vi "read_plc_global.vi"() -> ()   [LabVIEW 2011]
panel:
  out "Error in AO PLCs":errorcluster
  out "Error in AI PLCs":errorcluster
  out "LB201_B230_SV201":string
  out "LB201_B230_SV401":string
  out "LB201_B230_ST902":string
  out "LB201_B230_ST901":string
  out "LB201_A213_ST902":string
  out "LB201_A213_ST901":string
  out "LB201_A235_SV401":string
  out "LB201_A235_SV201":string
  out "LB201_A235_ST902":string
  out "LB201_A235_ST901":string
  out "LB201_A225_SV401":string
  out "LB201_A225_SV201":string
  out "LB201_A225_ST902":string
  out "LB201_A225_ST901":string
  out "LB201_A213_SV201":string
  out "LB201_A213_ST401":string
  out "LB201_B230_GQ101":string
  out "LB201_B230_GT101":string
  out "LB201_B226_GT301":string
  out "LB201_A235_GQ101":string
  out "LB201_A235_GT101":string
  out "LB201_B230_GN501":string
  out "LB201_A235_GN501":string
  out "LB201_A225_GT101":string
  out "LB201_A225_GQ101":string
  out "LB201_A225_GN501":string
  out "LB201_A213_GT101":string
  out "LB201_A213_GQ101":string
  out "LB201_A213_GN501":string
  out "Deque error":errorcluster
  out "DataSocket error":errorcluster
  out "# Sent Data":u64
  in  "Version":string
  in  "UpTime":string
  in  "StartupTime":string
  in  "ElapsedTime":u32
  in  "Command":string
  # "OPC Server Status"
  # "AI PLCs"
  # "AO PLCs"
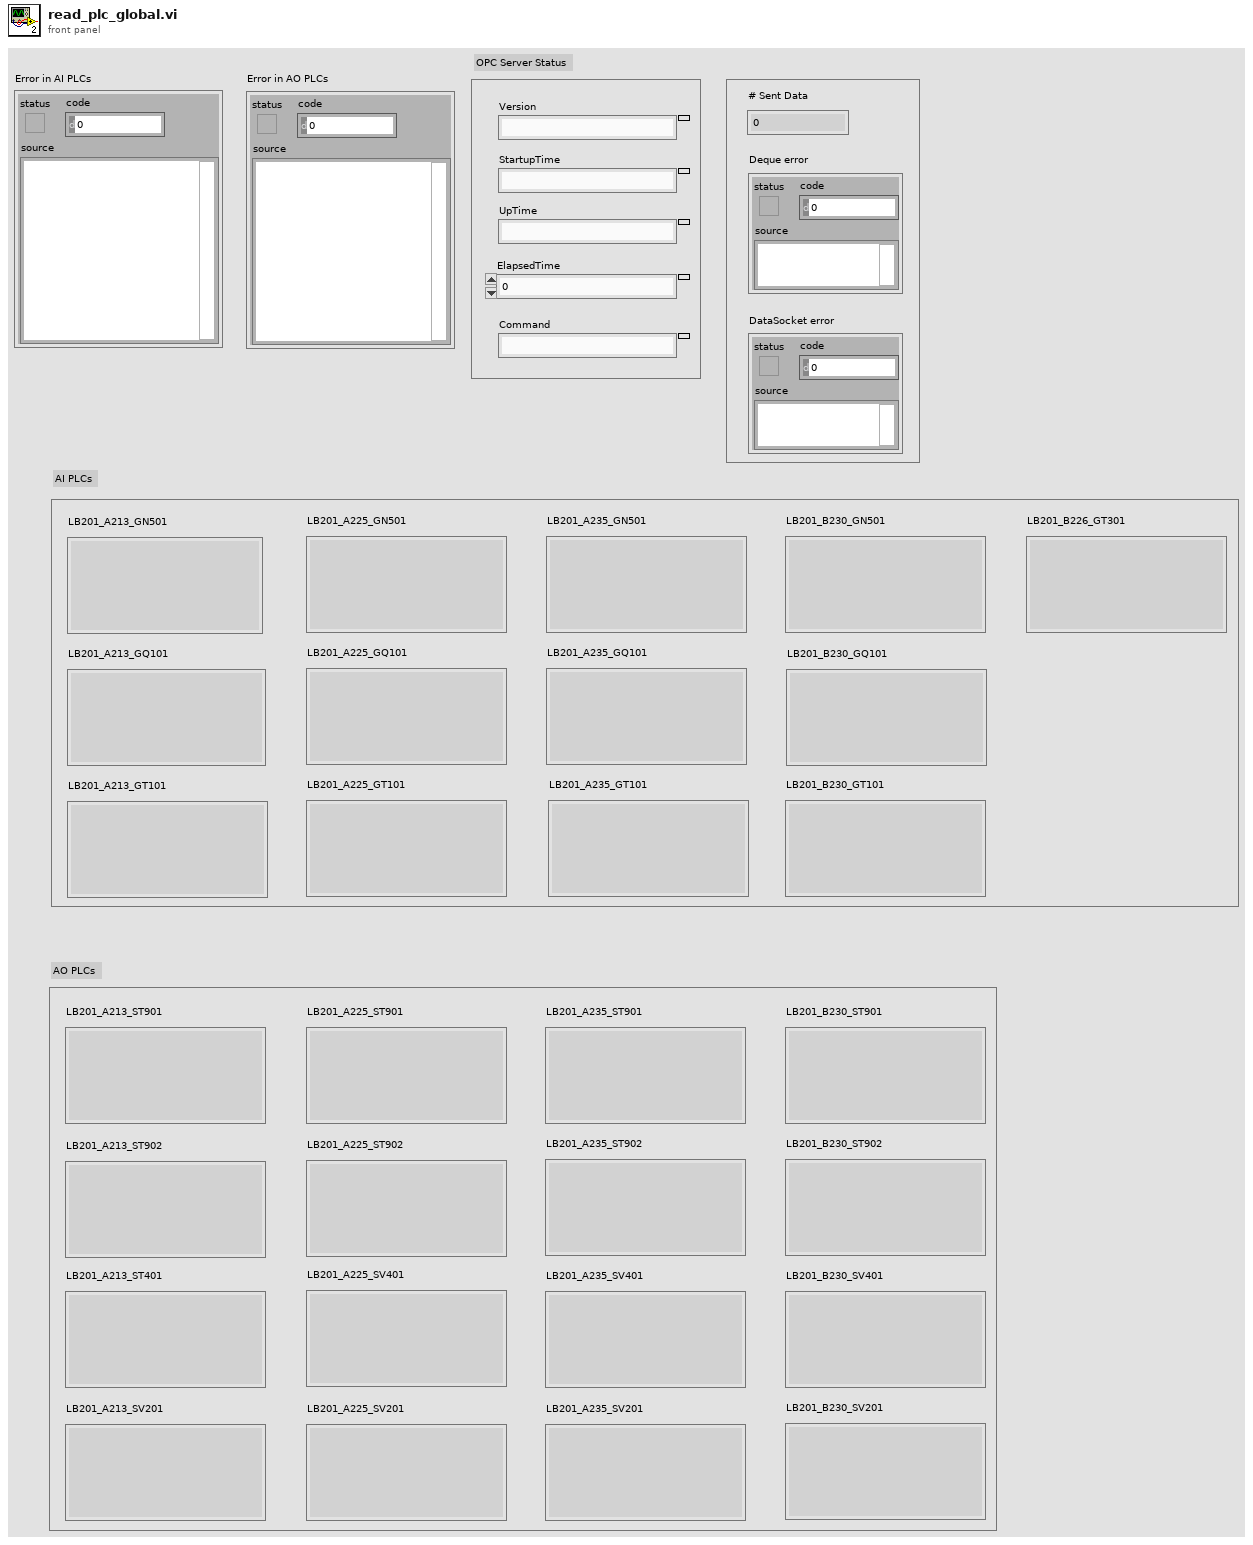
[diagram p1: front panel]
types:
  T1 = enum16{"Read", "Write", "ReadWrite", "BufferedRead", "BufferedReadWrite"}
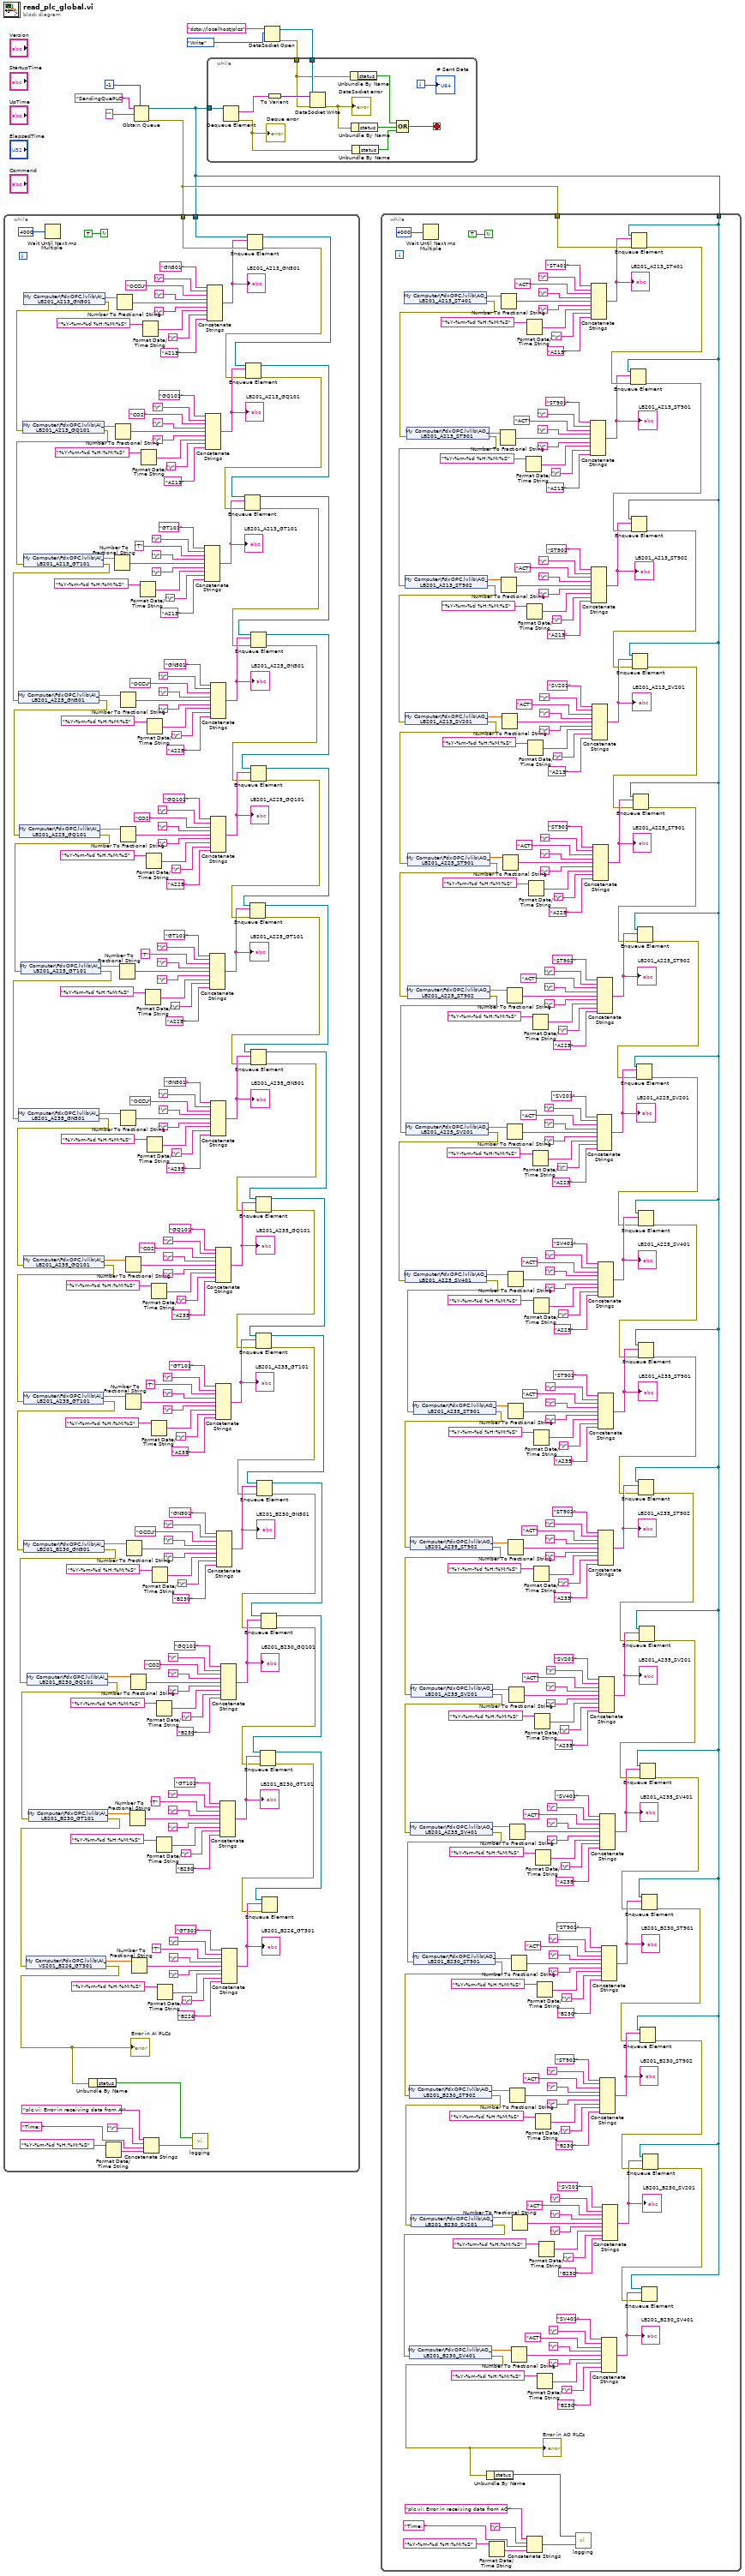
[diagram p0: block diagram]
diagram:
  n1 = Obtain Queue(max queue size (-1, unlimited)=-1, name (unnamed)="SendingQuePLC", element data type="") -> (queue out=w1:refnum<queue>, error out=w2:errorcluster)  [unwired: 2 in, 1 out]
  n2 = while {
    tunnel: w2 -> [w212]
    tunnel: w1 -> [w211]
    stop <- TRUE continue-if-true
    n3 = shared-variable "My Computer\\FdxOPC.lvlib\\AI_LB201_A213_GN501"() -> (w172:sgl, error out=w29:errorcluster)  [unwired: 1 in]
    n4 = shared-variable "My Computer\\FdxOPC.lvlib\\AI_LB201_A213_GQ101"(error in=w29) -> (w171:sgl, error out=w28:errorcluster)
    n5 = shared-variable "My Computer\\FdxOPC.lvlib\\AI_LB201_A213_GT101"(error in=w28) -> (w170:sgl, error out=w27:errorcluster)
    n6 = shared-variable "My Computer\\FdxOPC.lvlib\\AI_LB201_A225_GN501"(error in=w27) -> (w59:sgl, error out=w26:errorcluster)
    n7 = shared-variable "My Computer\\FdxOPC.lvlib\\AI_LB201_A225_GQ101"(error in=w26) -> (w56:sgl, error out=w25:errorcluster)
    n8 = shared-variable "My Computer\\FdxOPC.lvlib\\AI_LB201_A225_GT101"(error in=w25) -> (w55:sgl, error out=w24:errorcluster)
    n9 = shared-variable "My Computer\\FdxOPC.lvlib\\AI_LB201_A235_GN501"(error in=w24) -> (w54:sgl, error out=w23:errorcluster)
    n10 = shared-variable "My Computer\\FdxOPC.lvlib\\AI_LB201_A235_GQ101"(error in=w23) -> (w53:sgl, error out=w22:errorcluster)
    n11 = shared-variable "My Computer\\FdxOPC.lvlib\\AI_LB201_A235_GT101"(error in=w22) -> (w52:sgl, error out=w21:errorcluster)
    n12 = shared-variable "My Computer\\FdxOPC.lvlib\\AI_LB201_B230_GN501"(error in=w21) -> (w51:sgl, error out=w20:errorcluster)
    n13 = shared-variable "My Computer\\FdxOPC.lvlib\\AI_LB201_B230_GQ101"(error in=w20) -> (w50:sgl, error out=w19:errorcluster)
    n14 = shared-variable "My Computer\\FdxOPC.lvlib\\AI_LB201_B230_GT101"(error in=w19) -> (w49:sgl, error out=w18:errorcluster)
    n15 = shared-variable "My Computer\\FdxOPC.lvlib\\AI_VS201_B226_GT301"(error in=w18) -> (w48:sgl, error out=w17:errorcluster)
    "Error in AI PLCs" <- w17
    n16 = Wait Until Next ms Multiple(millisecond multiple=u32 4000) -> ()  [unwired: 1 out]
    n17 = Unbundle By Name(w17) -> ("status"=w10:bool)
    n18 = Format Date/Time String(time format string (%c)="%Y-%m-%d %H:%M:%S") -> (date/time string=w12:string)  [unwired: 2 in]
    n19 = Number To Fractional String(number=w170) -> (F-format string=w183:string)  [unwired: 3 in]
    n20 = Number To Fractional String(number=w171) -> (F-format string=w192:string)  [unwired: 3 in]
    n21 = Number To Fractional String(number=w172) -> (F-format string=w205:string)  [unwired: 3 in]
    n22 = Number To Fractional String(number=w55) -> (F-format string=w143:string)  [unwired: 3 in]
    n23 = Number To Fractional String(number=w56) -> (F-format string=w152:string)  [unwired: 3 in]
    n24 = Number To Fractional String(number=w59) -> (F-format string=w165:string)  [unwired: 3 in]
    n25 = Number To Fractional String(number=w54) -> (F-format string=w130:string)  [unwired: 3 in]
    n26 = Number To Fractional String(number=w52) -> (F-format string=w108:string)  [unwired: 3 in]
    n27 = Number To Fractional String(number=w53) -> (F-format string=w99:string)  [unwired: 3 in]
    n28 = Number To Fractional String(number=w51) -> (F-format string=w121:string)  [unwired: 3 in]
    n29 = Number To Fractional String(number=w49) -> (F-format string=w77:string)  [unwired: 3 in]
    n30 = Number To Fractional String(number=w50) -> (F-format string=w86:string)  [unwired: 3 in]
    n31 = Number To Fractional String(number=w48) -> (F-format string=w64:string)  [unwired: 3 in]
    n32 = Format Date/Time String(time format string (%c)="%Y-%m-%d %H:%M:%S") -> (date/time string=w182:string)  [unwired: 2 in]
    n33 = Format Date/Time String(time format string (%c)="%Y-%m-%d %H:%M:%S") -> (date/time string=w193:string)  [unwired: 2 in]
    n34 = Format Date/Time String(time format string (%c)="%Y-%m-%d %H:%M:%S") -> (date/time string=w204:string)  [unwired: 2 in]
    n35 = Concatenate Strings("plc.vi: Error in receiving data from AI", "\r", "Time: ", w12) -> (w13:string)
    n36 = Format Date/Time String(time format string (%c)="%Y-%m-%d %H:%M:%S") -> (date/time string=w142:string)  [unwired: 2 in]
    n37 = Format Date/Time String(time format string (%c)="%Y-%m-%d %H:%M:%S") -> (date/time string=w153:string)  [unwired: 2 in]
    n38 = Format Date/Time String(time format string (%c)="%Y-%m-%d %H:%M:%S") -> (date/time string=w164:string)  [unwired: 2 in]
    n39 = Format Date/Time String(time format string (%c)="%Y-%m-%d %H:%M:%S") -> (date/time string=w131:string)  [unwired: 2 in]
    n40 = Format Date/Time String(time format string (%c)="%Y-%m-%d %H:%M:%S") -> (date/time string=w109:string)  [unwired: 2 in]
    n41 = Format Date/Time String(time format string (%c)="%Y-%m-%d %H:%M:%S") -> (date/time string=w98:string)  [unwired: 2 in]
    n42 = Format Date/Time String(time format string (%c)="%Y-%m-%d %H:%M:%S") -> (date/time string=w120:string)  [unwired: 2 in]
    n43 = Format Date/Time String(time format string (%c)="%Y-%m-%d %H:%M:%S") -> (date/time string=w76:string)  [unwired: 2 in]
    n44 = Format Date/Time String(time format string (%c)="%Y-%m-%d %H:%M:%S") -> (date/time string=w87:string)  [unwired: 2 in]
    n45 = Format Date/Time String(time format string (%c)="%Y-%m-%d %H:%M:%S") -> (date/time string=w65:string)  [unwired: 2 in]
    n46 = call "logging.vi"("Body"=w13, "Enable"=w10) -> ()  [unwired: 1 in]
    n47 = Concatenate Strings("GT101" ("string"), "\r", "T" ("string"), "\r", w183, "\r", w182, "\r", "A213") -> (w186:string)
    "LB201_A213_GT101" <- w186
    n48 = Concatenate Strings("GQ101" ("string"), "\r", "CO2" ("string"), "\r", w192, "\r", w193, "\r", "A213") -> (w189:string)
    "LB201_A213_GQ101" <- w189
    n49 = Concatenate Strings("GN501" ("string"), "\r", "OCCU" ("string"), "\r", w205, "\r", w204, "\r", "A213") -> (w210:string)
    "LB201_A213_GN501" <- w210
    n50 = Concatenate Strings("GT101" ("string"), "\r", "T" ("string"), "\r", w143, "\r", w142, "\r", "A225") -> (w146:string)
    "LB201_A225_GT101" <- w146
    n51 = Concatenate Strings("GQ101" ("string"), "\r", "CO2" ("string"), "\r", w152, "\r", w153, "\r", "A225") -> (w149:string)
    "LB201_A225_GQ101" <- w149
    n52 = Concatenate Strings("GN501" ("string"), "\r", "OCCU" ("string"), "\r", w165, "\r", w164, "\r", "A225") -> (w168:string)
    "LB201_A225_GN501" <- w168
    n53 = Concatenate Strings("GN501" ("string"), "\r", "OCCU" ("string"), "\r", w130, "\r", w131, "\r", "A235") -> (w127:string)
    "LB201_A235_GN501" <- w127
    n54 = Concatenate Strings("GT101" ("string"), "\r", "T" ("string"), "\r", w108, "\r", w109, "\r", "A235") -> (w105:string)
    "LB201_A235_GT101" <- w105
    n55 = Concatenate Strings("GQ101" ("string"), "\r", "CO2" ("string"), "\r", w99, "\r", w98, "\r", "A235") -> (w102:string)
    "LB201_A235_GQ101" <- w102
    n56 = Concatenate Strings("GN501" ("string"), "\r", "OCCU" ("string"), "\r", w121, "\r", w120, "\r", "B230") -> (w124:string)
    "LB201_B230_GN501" <- w124
    n57 = Concatenate Strings("GT101" ("string"), "\r", "T" ("string"), "\r", w77, "\r", w76, "\r", "B230") -> (w80:string)
    "LB201_B230_GT101" <- w80
    n58 = Concatenate Strings("GQ101" ("string"), "\r", "CO2" ("string"), "\r", w86, "\r", w87, "\r", "B230") -> (w83:string)
    "LB201_B230_GQ101" <- w83
    n59 = Concatenate Strings("GT301" ("string"), "\r", "T" ("string"), "\r", w64, "\r", w65, "\r", "B226") -> (w61:string)
    "LB201_B226_GT301" <- w61
    n60 = Enqueue Element(queue=w211, element=w210, error in (no error)=w212) -> (queue out=w176:refnum<queue>, error out=w174:errorcluster)  [unwired: 1 in, 1 out]
    n61 = Enqueue Element(queue=w176, element=w189, error in (no error)=w174) -> (queue out=w175:refnum<queue>, error out=w173:errorcluster)  [unwired: 1 in, 1 out]
    n62 = Enqueue Element(queue=w175, element=w186, error in (no error)=w173) -> (queue out=w58:refnum<queue>, error out=w57:errorcluster)  [unwired: 1 in, 1 out]
    n63 = Enqueue Element(queue=w58, element=w168, error in (no error)=w57) -> (queue out=w47:refnum<queue>, error out=w46:errorcluster)  [unwired: 1 in, 1 out]
    n64 = Enqueue Element(queue=w47, element=w149, error in (no error)=w46) -> (queue out=w45:refnum<queue>, error out=w44:errorcluster)  [unwired: 1 in, 1 out]
    n65 = Enqueue Element(queue=w45, element=w146, error in (no error)=w44) -> (queue out=w43:refnum<queue>, error out=w42:errorcluster)  [unwired: 1 in, 1 out]
    n66 = Enqueue Element(queue=w43, element=w127, error in (no error)=w42) -> (queue out=w41:refnum<queue>, error out=w40:errorcluster)  [unwired: 1 in, 1 out]
    n67 = Enqueue Element(queue=w41, element=w102, error in (no error)=w40) -> (queue out=w39:refnum<queue>, error out=w38:errorcluster)  [unwired: 1 in, 1 out]
    n68 = Enqueue Element(queue=w39, element=w105, error in (no error)=w38) -> (queue out=w37:refnum<queue>, error out=w36:errorcluster)  [unwired: 1 in, 1 out]
    n69 = Enqueue Element(queue=w37, element=w124, error in (no error)=w36) -> (queue out=w35:refnum<queue>, error out=w34:errorcluster)  [unwired: 1 in, 1 out]
    n70 = Enqueue Element(queue=w35, element=w83, error in (no error)=w34) -> (queue out=w33:refnum<queue>, error out=w32:errorcluster)  [unwired: 1 in, 1 out]
    n71 = Enqueue Element(queue=w33, element=w80, error in (no error)=w32) -> (queue out=w31:refnum<queue>, error out=w30:errorcluster)  [unwired: 1 in, 1 out]
    n72 = Enqueue Element(queue=w31, element=w61, error in (no error)=w30) -> ()  [unwired: 1 in, 3 out]
  }
  n73 = DataSocket Open(10:T1."Write" ("mode"), 11:"dstp://localhost/plcs" ("URL 3")) -> (0:w4:errorcluster, 3:w5:refnum<k13>)  [unwired: 2 in]
  n74 = while {
    tunnel: w1 -> [w225]
    tunnel: w5 -> [w224]
    tunnel: w4 -> [w217]
    i -> [w214]
    stop <- w215 stop-if-true
    n75 = Dequeue Element(queue=w225) -> (element=w222:string, error out=w221:errorcluster)  [unwired: 2 in, 2 out]
    "Deque error" <- w221
    n76 = To Variant(anything=w222) -> (Variant=w223:variant)
    n77 = DataSocket Write(8:w217, 10:w223, 11:w224) -> (0:w220:errorcluster)  [unwired: 3 out]
    "DataSocket error" <- w220
    n78 = Unbundle By Name(w217) -> ("status"=w216:bool)
    n79 = Unbundle By Name(w220) -> ("status"=w219:bool)
    n80 = Unbundle By Name(w221) -> ("status"=w218:bool)
    n81 = Compound Arithmetic op=OR(w216, w219, w218) -> (w215:bool)
    "# Sent Data" <- w214
  }
  n82 = while {
    tunnel: w2 -> [w327]
    tunnel: w1 -> [w226]
    stop <- TRUE continue-if-true
    n83 = shared-variable "My Computer\\FdxOPC.lvlib\\AO_LB201_A213_ST401"() -> (w326:sgl, error out=w249:errorcluster)  [unwired: 1 in]
    n84 = shared-variable "My Computer\\FdxOPC.lvlib\\AO_LB201_A213_ST901"(error in=w249) -> (w325:sgl, error out=w248:errorcluster)
    n85 = shared-variable "My Computer\\FdxOPC.lvlib\\AO_LB201_A213_ST902"(error in=w248) -> (w324:sgl, error out=w247:errorcluster)
    n86 = shared-variable "My Computer\\FdxOPC.lvlib\\AO_LB201_A213_SV201"(error in=w247) -> (w323:sgl, error out=w246:errorcluster)
    n87 = shared-variable "My Computer\\FdxOPC.lvlib\\AO_LB201_A225_ST901"(error in=w246) -> (w319:sgl, error out=w245:errorcluster)
    n88 = shared-variable "My Computer\\FdxOPC.lvlib\\AO_LB201_A225_ST902"(error in=w245) -> (w318:sgl, error out=w244:errorcluster)
    n89 = shared-variable "My Computer\\FdxOPC.lvlib\\AO_LB201_A225_SV201"(error in=w244) -> (w317:sgl, error out=w243:errorcluster)
    n90 = shared-variable "My Computer\\FdxOPC.lvlib\\AO_LB201_A225_SV401"(error in=w243) -> (w316:sgl, error out=w242:errorcluster)
    n91 = shared-variable "My Computer\\FdxOPC.lvlib\\AO_LB201_A235_ST901"(error in=w242) -> (w309:sgl, error out=w241:errorcluster)
    n92 = shared-variable "My Computer\\FdxOPC.lvlib\\AO_LB201_A235_ST902"(error in=w241) -> (w308:sgl, error out=w240:errorcluster)
    n93 = shared-variable "My Computer\\FdxOPC.lvlib\\AO_LB201_A235_SV201"(error in=w240) -> (w307:sgl, error out=w239:errorcluster)
    n94 = shared-variable "My Computer\\FdxOPC.lvlib\\AO_LB201_A235_SV401"(error in=w239) -> (w306:sgl, error out=w238:errorcluster)
    n95 = shared-variable "My Computer\\FdxOPC.lvlib\\AO_LB201_B230_ST901"(error in=w238) -> (w258:sgl, error out=w237:errorcluster)
    n96 = shared-variable "My Computer\\FdxOPC.lvlib\\AO_LB201_B230_ST902"(error in=w237) -> (w257:sgl, error out=w236:errorcluster)
    n97 = shared-variable "My Computer\\FdxOPC.lvlib\\AO_LB201_B230_SV201"(error in=w236) -> (w256:sgl, error out=w235:errorcluster)
    n98 = shared-variable "My Computer\\FdxOPC.lvlib\\AO_LB201_B230_SV401"(error in=w235) -> (w255:sgl, error out=w234:errorcluster)
    "Error in AO PLCs" <- w234
    n99 = Wait Until Next ms Multiple(millisecond multiple=u32 4000) -> ()  [unwired: 1 out]
    n100 = Unbundle By Name(w234) -> ("status"=w227:bool)
    n101 = Format Date/Time String(time format string (%c)="%Y-%m-%d %H:%M:%S") -> (date/time string=w229:string)  [unwired: 2 in]
    n102 = Number To Fractional String(number=w325) -> (F-format string=w443:string)  [unwired: 3 in]
    n103 = Number To Fractional String(number=w326) -> (F-format string=w435:string)  [unwired: 3 in]
    n104 = Number To Fractional String(number=w324) -> (F-format string=w456:string)  [unwired: 3 in]
    n105 = Number To Fractional String(number=w323) -> (F-format string=w422:string)  [unwired: 3 in]
    n106 = Number To Fractional String(number=w319) -> (F-format string=w334:string)  [unwired: 3 in]
    n107 = Number To Fractional String(number=w317) -> (F-format string=w356:string)  [unwired: 3 in]
    n108 = Number To Fractional String(number=w318) -> (F-format string=w347:string)  [unwired: 3 in]
    n109 = Number To Fractional String(number=w316) -> (F-format string=w369:string)  [unwired: 3 in]
    n110 = Number To Fractional String(number=w308) -> (F-format string=w391:string)  [unwired: 3 in]
    n111 = Number To Fractional String(number=w309) -> (F-format string=w400:string)  [unwired: 3 in]
    n112 = Number To Fractional String(number=w307) -> (F-format string=w378:string)  [unwired: 3 in]
    n113 = Number To Fractional String(number=w306) -> (F-format string=w413:string)  [unwired: 3 in]
    n114 = Number To Fractional String(number=w257) -> (F-format string=w286:string)  [unwired: 3 in]
    n115 = Number To Fractional String(number=w258) -> (F-format string=w295:string)  [unwired: 3 in]
    n116 = Number To Fractional String(number=w255) -> (F-format string=w273:string)  [unwired: 3 in]
    n117 = Number To Fractional String(number=w256) -> (F-format string=w265:string)  [unwired: 3 in]
    n118 = Format Date/Time String(time format string (%c)="%Y-%m-%d %H:%M:%S") -> (date/time string=w444:string)  [unwired: 2 in]
    n119 = Format Date/Time String(time format string (%c)="%Y-%m-%d %H:%M:%S") -> (date/time string=w434:string)  [unwired: 2 in]
    n120 = Concatenate Strings("plc.vi: Error in receiving data from AO", "\r", "Time: ", w229) -> (w230:string)
    n121 = Format Date/Time String(time format string (%c)="%Y-%m-%d %H:%M:%S") -> (date/time string=w455:string)  [unwired: 2 in]
    n122 = Format Date/Time String(time format string (%c)="%Y-%m-%d %H:%M:%S") -> (date/time string=w423:string)  [unwired: 2 in]
    n123 = Format Date/Time String(time format string (%c)="%Y-%m-%d %H:%M:%S") -> (date/time string=w335:string)  [unwired: 2 in]
    n124 = Format Date/Time String(time format string (%c)="%Y-%m-%d %H:%M:%S") -> (date/time string=w357:string)  [unwired: 2 in]
    n125 = Format Date/Time String(time format string (%c)="%Y-%m-%d %H:%M:%S") -> (date/time string=w346:string)  [unwired: 2 in]
    n126 = Format Date/Time String(time format string (%c)="%Y-%m-%d %H:%M:%S") -> (date/time string=w368:string)  [unwired: 2 in]
    n127 = Format Date/Time String(time format string (%c)="%Y-%m-%d %H:%M:%S") -> (date/time string=w390:string)  [unwired: 2 in]
    n128 = Format Date/Time String(time format string (%c)="%Y-%m-%d %H:%M:%S") -> (date/time string=w401:string)  [unwired: 2 in]
    n129 = Format Date/Time String(time format string (%c)="%Y-%m-%d %H:%M:%S") -> (date/time string=w379:string)  [unwired: 2 in]
    n130 = Format Date/Time String(time format string (%c)="%Y-%m-%d %H:%M:%S") -> (date/time string=w412:string)  [unwired: 2 in]
    n131 = Format Date/Time String(time format string (%c)="%Y-%m-%d %H:%M:%S") -> (date/time string=w285:string)  [unwired: 2 in]
    n132 = Format Date/Time String(time format string (%c)="%Y-%m-%d %H:%M:%S") -> (date/time string=w296:string)  [unwired: 2 in]
    n133 = Format Date/Time String(time format string (%c)="%Y-%m-%d %H:%M:%S") -> (date/time string=w274:string)  [unwired: 2 in]
    n134 = Format Date/Time String(time format string (%c)="%Y-%m-%d %H:%M:%S") -> (date/time string=w264:string)  [unwired: 2 in]
    n135 = call "logging.vi"("Body"=w230, "Enable"=w227) -> ()  [unwired: 1 in]
    n136 = Concatenate Strings("ST901" ("string"), "\r", "ACT" ("string"), "\r", w443, "\r", w444, "\r", "A213") -> (w311:string)
    "LB201_A213_ST901" <- w311
    n137 = Concatenate Strings("ST401" ("string"), "\r", "ACT" ("string"), "\r", w435, "\r", w434, "\r", "A213") -> (w438:string)
    "LB201_A213_ST401" <- w438
    n138 = Concatenate Strings("ST902" ("string"), "\r", "ACT" ("string"), "\r", w456, "\r", w455, "\r", "A213") -> (w310:string)
    "LB201_A213_ST902" <- w310
    n139 = Concatenate Strings("SV201" ("string"), "\r", "ACT" ("string"), "\r", w422, "\r", w423, "\r", "A213") -> (w419:string)
    "LB201_A213_SV201" <- w419
    n140 = Concatenate Strings("ST901" ("string"), "\r", "ACT" ("string"), "\r", w334, "\r", w335, "\r", "A225") -> (w331:string)
    "LB201_A225_ST901" <- w331
    n141 = Concatenate Strings("SV201" ("string"), "\r", "ACT" ("string"), "\r", w356, "\r", w357, "\r", "A225") -> (w353:string)
    "LB201_A225_SV201" <- w353
    n142 = Concatenate Strings("ST902" ("string"), "\r", "ACT" ("string"), "\r", w347, "\r", w346, "\r", "A225") -> (w350:string)
    "LB201_A225_ST902" <- w350
    n143 = Concatenate Strings("SV401" ("string"), "\r", "ACT" ("string"), "\r", w369, "\r", w368, "\r", "A225") -> (w372:string)
    "LB201_A225_SV401" <- w372
    n144 = Concatenate Strings("ST902" ("string"), "\r", "ACT" ("string"), "\r", w391, "\r", w390, "\r", "A235") -> (w394:string)
    "LB201_A235_ST902" <- w394
    n145 = Concatenate Strings("ST901" ("string"), "\r", "ACT" ("string"), "\r", w400, "\r", w401, "\r", "A235") -> (w397:string)
    "LB201_A235_ST901" <- w397
    n146 = Concatenate Strings("SV201" ("string"), "\r", "ACT" ("string"), "\r", w378, "\r", w379, "\r", "A235") -> (w375:string)
    "LB201_A235_SV201" <- w375
    n147 = Concatenate Strings("SV401" ("string"), "\r", "ACT" ("string"), "\r", w413, "\r", w412, "\r", "A235") -> (w416:string)
    "LB201_A235_SV401" <- w416
    n148 = Concatenate Strings("ST902" ("string"), "\r", "ACT" ("string"), "\r", w286, "\r", w285, "\r", "B230") -> (w289:string)
    "LB201_B230_ST902" <- w289
    n149 = Concatenate Strings("ST901" ("string"), "\r", "ACT" ("string"), "\r", w295, "\r", w296, "\r", "B230") -> (w292:string)
    "LB201_B230_ST901" <- w292
    n150 = Concatenate Strings("SV401" ("string"), "\r", "ACT" ("string"), "\r", w273, "\r", w274, "\r", "B230") -> (w270:string)
    "LB201_B230_SV401" <- w270
    n151 = Concatenate Strings("SV201" ("string"), "\r", "ACT" ("string"), "\r", w265, "\r", w264, "\r", "B230") -> (w252:string)
    "LB201_B230_SV201" <- w252
    n152 = Enqueue Element(queue=w226, element=w438, error in (no error)=w327) -> (error out=w322:errorcluster)  [unwired: 1 in, 2 out]
    n153 = Enqueue Element(queue=w226, element=w311, error in (no error)=w322) -> (error out=w321:errorcluster)  [unwired: 1 in, 2 out]
    n154 = Enqueue Element(queue=w226, element=w310, error in (no error)=w321) -> (error out=w320:errorcluster)  [unwired: 1 in, 2 out]
    n155 = Enqueue Element(queue=w226, element=w419, error in (no error)=w320) -> (error out=w315:errorcluster)  [unwired: 1 in, 2 out]
    n156 = Enqueue Element(queue=w226, element=w331, error in (no error)=w315) -> (error out=w314:errorcluster)  [unwired: 1 in, 2 out]
    n157 = Enqueue Element(queue=w226, element=w350, error in (no error)=w314) -> (error out=w313:errorcluster)  [unwired: 1 in, 2 out]
    n158 = Enqueue Element(queue=w226, element=w353, error in (no error)=w313) -> (error out=w312:errorcluster)  [unwired: 1 in, 2 out]
    n159 = Enqueue Element(queue=w226, element=w372, error in (no error)=w312) -> (error out=w305:errorcluster)  [unwired: 1 in, 2 out]
    n160 = Enqueue Element(queue=w226, element=w397, error in (no error)=w305) -> (error out=w304:errorcluster)  [unwired: 1 in, 2 out]
    n161 = Enqueue Element(queue=w226, element=w394, error in (no error)=w304) -> (error out=w303:errorcluster)  [unwired: 1 in, 2 out]
    n162 = Enqueue Element(queue=w226, element=w375, error in (no error)=w303) -> (error out=w302:errorcluster)  [unwired: 1 in, 2 out]
    n163 = Enqueue Element(queue=w226, element=w416, error in (no error)=w302) -> (error out=w254:errorcluster)  [unwired: 1 in, 2 out]
    n164 = Enqueue Element(queue=w226, element=w292, error in (no error)=w254) -> (error out=w253:errorcluster)  [unwired: 1 in, 2 out]
    n165 = Enqueue Element(queue=w226, element=w289, error in (no error)=w253) -> (error out=w251:errorcluster)  [unwired: 1 in, 2 out]
    n166 = Enqueue Element(queue=w226, element=w252, error in (no error)=w251) -> (error out=w250:errorcluster)  [unwired: 1 in, 2 out]
    n167 = Enqueue Element(queue=w226, element=w270, error in (no error)=w250) -> ()  [unwired: 1 in, 3 out]
  }
